vi "SP_Production_Count_DayWise_1.vi"(8 "error in (no error)":errorcluster) -> (0 "error out":errorcluster)   [LabVIEW 2017]
uses:
  <vilib>/Math Plots/3D Math Plots/3D Pie/3D Pie XCtrl/3D Pie.xctl
  <vilib>/addons/database/Connection.llb/DB Tools Open Connec (Path).vi
  <vilib>/addons/database/Connection.llb/Conn Execute.vi
  <vilib>/addons/database/Recordset.llb/Rec Fetch Recordset Data (R).vi
  <vilib>/addons/database/Recordset.llb/Rec Destroy - Connection.vi
  <vilib>/Math Plots/3D Math Plots/3D Pie/3D Pie Datatype/Public/Plot Helper (Vector).vi
  <vilib>/addons/database/NI_Database_API.lvlib
  <vilib>/Math Plots/3D Math Plots/3D Pie/3D Pie Datatype/3D Pie Datatype.lvclass
panel:
  out "Station size":i32
  in  "Tab Control":enum32{"Data", "Graph"}(tab)
  out "Table":string[][](table)
  out "3D Pie":refnum<class "3D Plot Datatype.lvclass">[](xcontrol)
  in  "To Date":timestamp format="%<%Y-%m-%d>T"
  out "Station Count":i32
  in  "Cancel Button - Archive":bool
  in  "Download 2":bool
  in  "Get Rport 2":bool
  in  "Shift":string(combo)
  in  "Station":string(combo)
  in  "From Date":timestamp format="%<%Y-%m-%d>T"
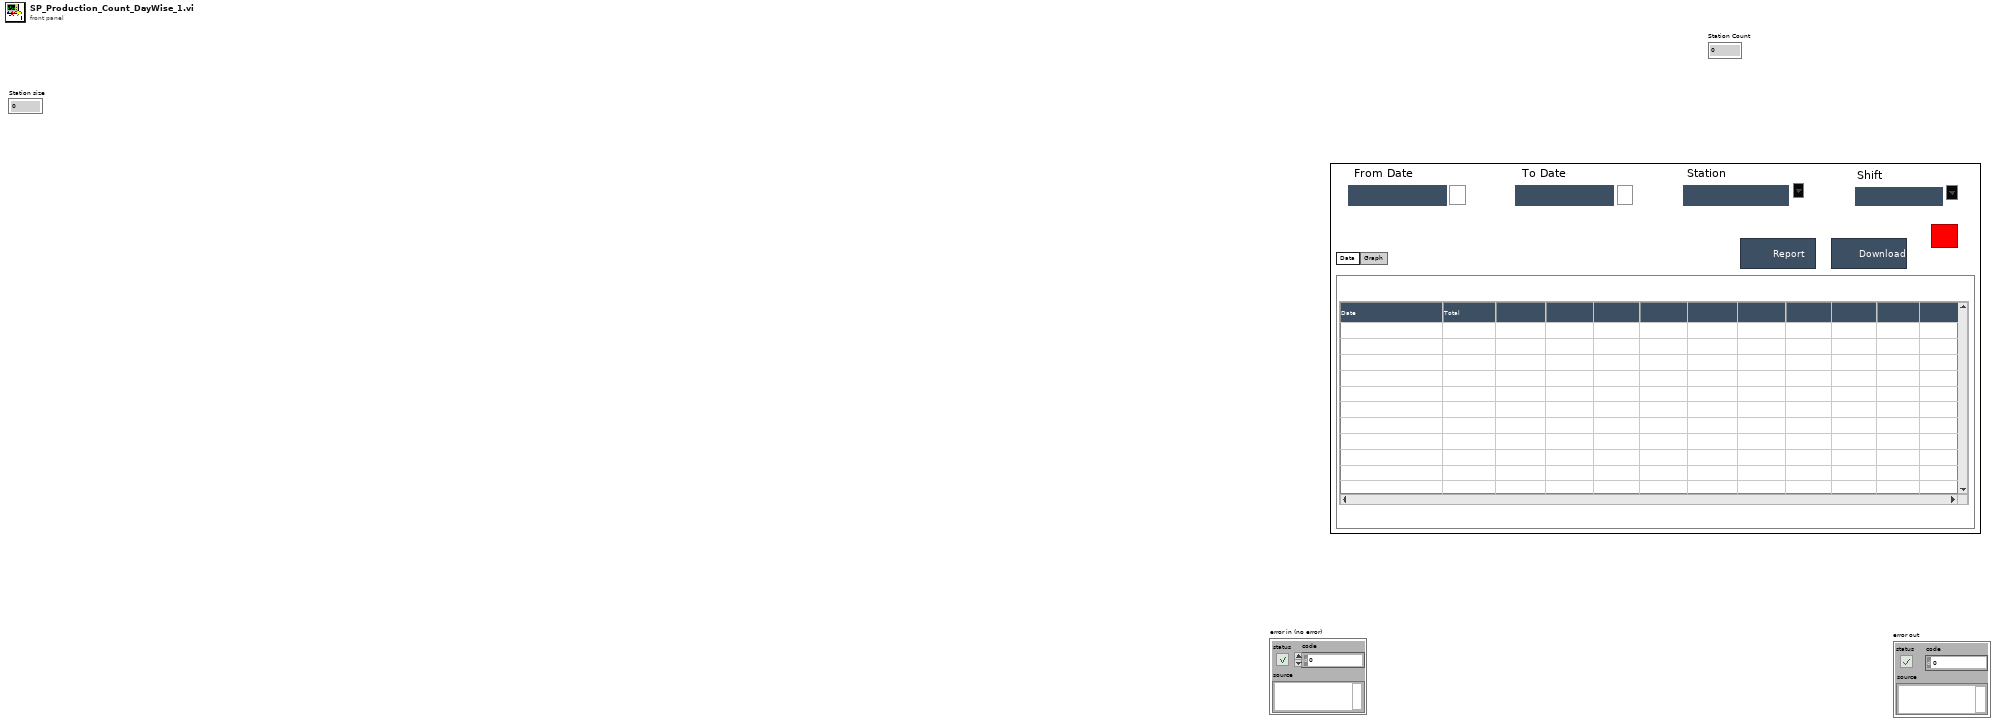
[diagram p1: front panel]
types:
  T1 = typedef "NI_Database_API.lvlib/Conn ObjectReference.ctl" = refnum<k1>
  T2 = typedef "NI_Database_API.lvlib/Rec ObjectReference.ctl" = refnum<k1>
  T3 = enum32{"invalid app kind", "Development System", "Run Time System", "Student Edition", "Embedded LabVIEW", "Evaluation", "Custom"}
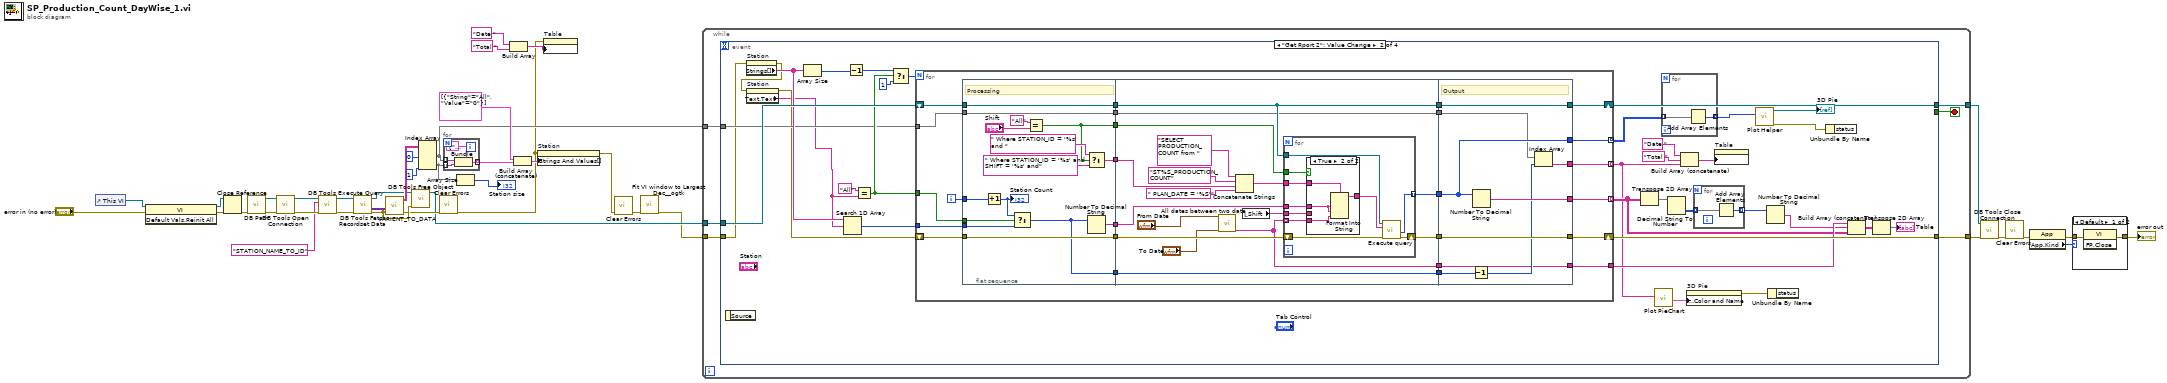
[diagram p0: block diagram]
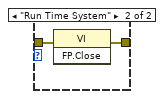
[diagram p2: hidden frame]
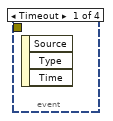
[diagram p3: hidden frame]
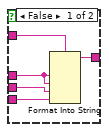
[diagram p4: hidden frame]
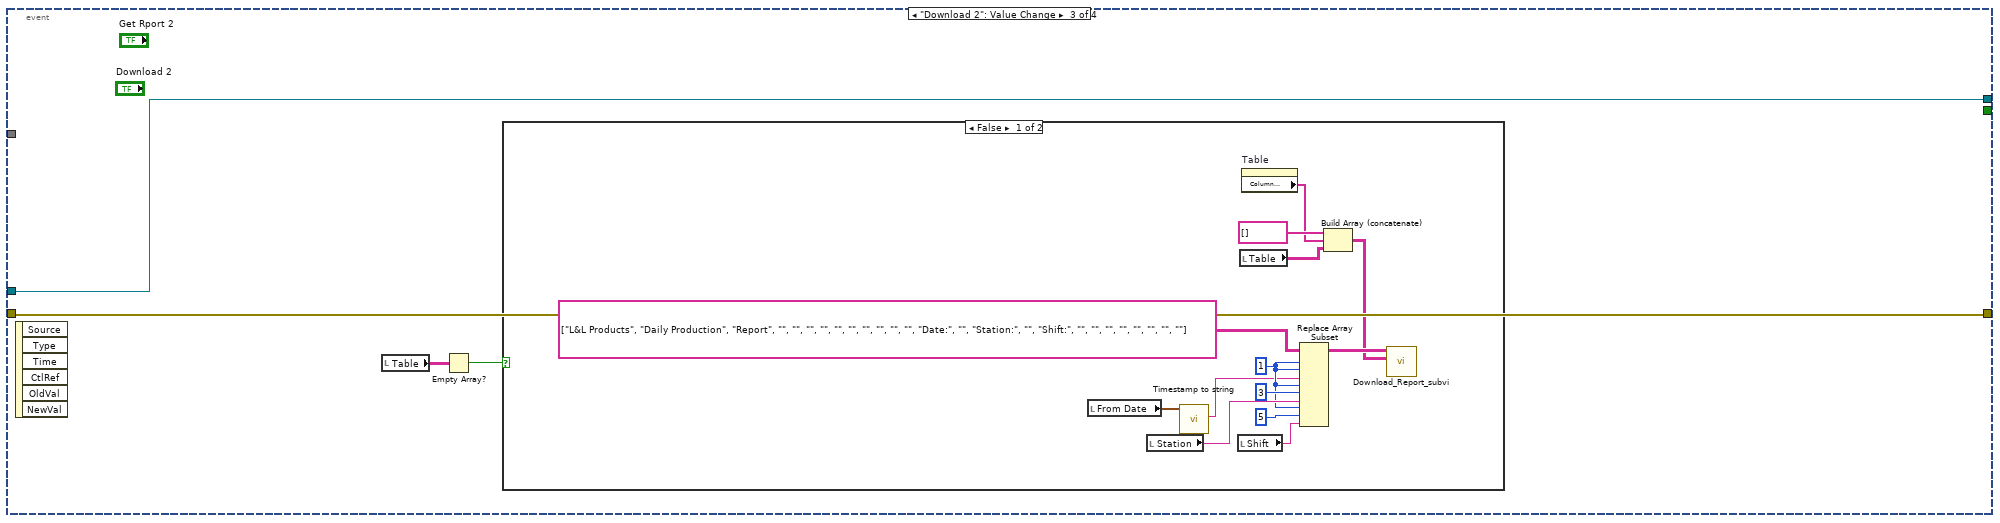
[diagram p5: hidden frame]
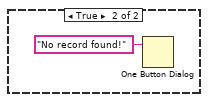
[diagram p6: hidden frame]
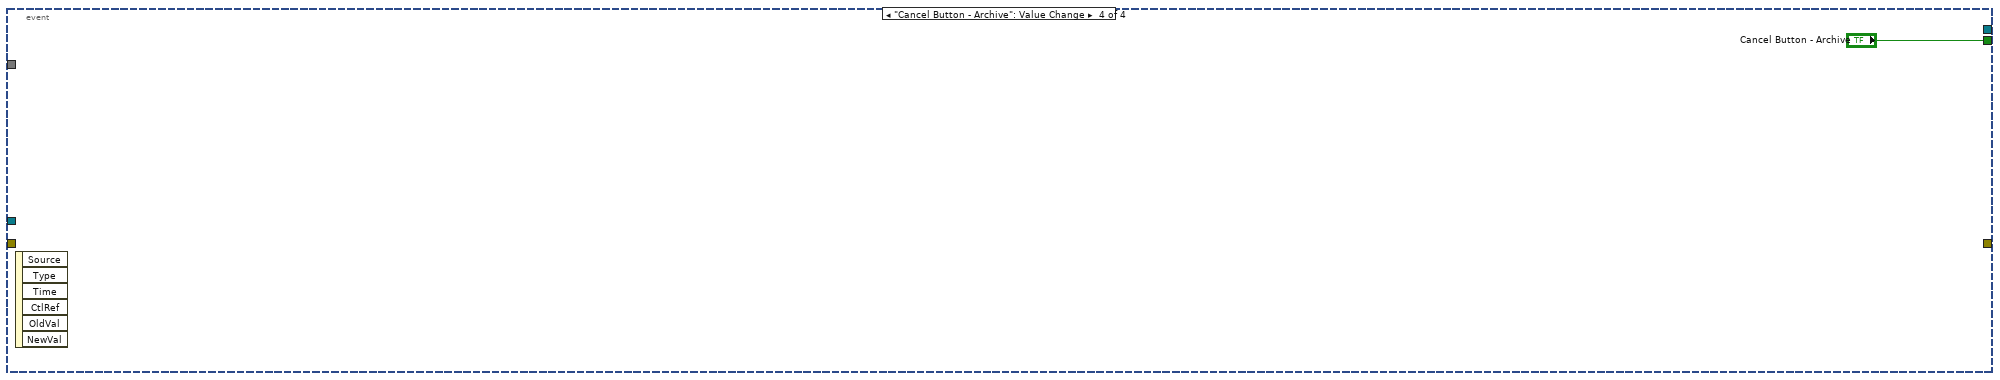
[diagram p7: hidden frame]
diagram:
  n1 = control-ref of="This VI"() -> (w32:refnum<vi>)
  n2 = invoke class="VI" method="Default Vals.Reinit All"(reference=w32, error in="error in (no error)") -> (reference out=w30:refnum<vi>, error out=w31:errorcluster)  [unwired: 1 in, 1 out]
  n3 = Close Reference(reference=w30, error in (no error)=w31) -> (error out=w29:errorcluster)
  n4 = call "DB Path.vi"("error in"=w29) -> ("error out"=w28:errorcluster, "DB Path"=w27:path)  [unwired: 9 in]
  n5 = call-poly <vilib>:"DB Tools Open Connection.vi"("error in (no error)"=w28, "connection information"=w27) -> ("error out"=w16:errorcluster, "connection reference"=w17:T1)  [unwired: 6 in]
  n6 = call-poly <vilib>:"DB Tools Execute Query.vi"("error in (no error)"=w16, "SQL query"="STATION_NAME_TO_ID", "connection reference"=w17) -> ("error out"=w25:errorcluster, "recordset reference"=w26:T2)  [unwired: 5 in]
  n7 = call-poly <vilib>:"DB Tools Fetch Recordset Data.vi"("error in (no error)"=w25, "recordset reference"=w26) -> ("error out"=w20:errorcluster, "recordset data"=w24:variant[][], "recordset reference out"=w18:T2)  [unwired: 3 in]
  n8 = call "VARIENT_TO_DATA.vi"("data"=w24, "error in (no error)"=w20) -> ("Table"=w21:string[][], "error out"=w19:errorcluster)  [unwired: 7 in]
  n9 = call-poly <vilib>:"DB Tools Free Object.vi"("error in (no error)"=w20, "recordset reference"=w18) -> ("connection reference"=w9:T1)  [unwired: 8 in, 1 out]
  n10 = Index Array(array=w21, index (col) #1=0 ("index (row)"), index (col) #2=1 ("index (col)")) -> (element #1=w5:string[], element #2=w11:string[])  [unwired: 2 in]
  n11 = call <vilib>:"Clear Errors.vi"("error in (no error)"=w19) -> ("error out"=w1:errorcluster)  [unwired: 5 in, 1 out]
  n12 = for {
    tunnel: w5 -> [w44] mode=indexing
    tunnel: w11 -> [w43] mode=indexing
    tunnel: [w41] -> w12 mode=indexing
    n13 = Bundle(cluster=cluster{"String":string, "Value":string} {"String"="", "Value"=""}, "String"=w44, "Value"=w43) -> (w41:cluster{"String":string, "Value":string})
  }
  n14 = Array Size(array=w11) -> (size(s)=→"Station size":i32)
  n15 = Build Array("Date ", "Total ") -> (w2:string[])
  n16 = Build Array (concatenate)(cluster{"String":string, "Value":string}[] [{"String"="All", "Value"="0"}] ("array"), w12) -> (w14:cluster{"String":string, "Value":string}[])
  n17 = property on="Station" class="CmbBox"(error in=w1, "Strings And Values[]"=w14) -> (error out=w7:errorcluster)  [unwired: 1 in, 1 out]
  n18 = property on="Table" class="Tbl (strict)"(error in=w1, "Column Headers[]"=w2) -> ()  [unwired: 1 in, 2 out]
  n19 = call <vilib>:"Clear Errors.vi"("error in (no error)"=w7) -> ("error out"=w8:errorcluster)  [unwired: 5 in, 1 out]
  n20 = call <userlib>:"Fit VI window to Largest Dec__ogtk.vi"("error in (no error)"=w8) -> ("error out"=w6:errorcluster)  [unwired: 5 in, 1 out]
  n21 = while {
    tunnel: w6 -> [w47]
    tunnel: w9 -> [w46]
    tunnel: [w49] -> w35
    tunnel: [w48] -> w34
    tunnel: w5 -> [w45]
    stop <- w50 stop-if-true
    n22 = event shown="[1] \"Get Rport 2\": Value Change" {
      selector: _ -> [_ _ _ _]
      dyn-events: _ -> [_ _ _ _]
      timeout: _ -> [_ _ _ _]
      tunnel: w46 -> [_ w84 w177 _]
      tunnel: [_ _ _ "Cancel Button - Archive"] -> w50
      tunnel: [_ w82 w176 _] -> w49
      tunnel: [_ w83 w177 _] -> w48
      tunnel: w47 -> [_ w53 w176 _]
      tunnel: w45 -> [_ w55 _ _]
      event Timeout {
        n23 = event-data() -> ()  [unwired: 1 in, 3 out]
      }
      event "Get Rport 2": Value Change {
        n24 = event-data() -> ()  [unwired: 1 in, 1 out]
        n25 = property on="Station" class="CmbBox"(error in=w53) -> (error out=w54:errorcluster, "Strings[]"=w63:string[])  [unwired: 1 in, 1 out]
        n26 = property on="Station" class="CmbBox"(error in=w54) -> (error out=w52:errorcluster, "Text.Text"=w51:string)  [unwired: 1 in, 1 out]
        n27 = Array Size(array=w63) -> (size(s)=w78:i32)
        n28 = Search 1D Array(1D array=w63, element=w51) -> (index of element=w75:i32)  [unwired: 1 in]
        n29 = Decrement(x=w78) -> (x-1=w77:i32)
        n30 = Equal?(x="All", y=w51) -> (x = y?=w76:bool)
        n31 = Select(t=w77, s=w76, f=1) -> (s? t:f=w80:i32)
        n32 = for {
          N: w80 -> [_]
          shift-right: [w106] -> w83
          shift-left: w84 -> [w113]
          shift-right: [w107] -> w82
          shift-left: w52 -> [w112]
          tunnel: w76 -> [w111]
          tunnel: w75 -> [w110]
          tunnel: [w108] -> w57 mode=indexing
          tunnel: [w98] -> w68 mode=indexing
          tunnel: [w97] -> w71
          tunnel: [w92] -> w59 mode=indexing
          tunnel: w55 -> [w89]
          i -> [w109]
          n33 = flat-sequence {
            tunnel: [w125] -> w105
            tunnel: [w126] -> w103
            tunnel: [w128] -> w101
            tunnel: [w127] -> w100
            tunnel: w109 -> [w120]
            tunnel: w110 -> [w121]
            tunnel: w111 -> [w122]
            tunnel: w112 -> [w125]
            tunnel: w113 -> [w126]
            tunnel: [w116] -> w95
            tunnel: [w115] -> w93
            tunnel: [w114] -> w90
            tunnel: w89 -> [w114]
            tunnel: w105 -> [w138]
            tunnel: [w137] -> w104
            tunnel: w103 -> [w139]
            tunnel: [w139] -> w102
            tunnel: w101 -> [w143]
            tunnel: w100 -> [w135]
            tunnel: [w136] -> w99
            tunnel: [w134] -> w96
            tunnel: w95 -> [w131]
            tunnel: [w130] -> w94
            tunnel: w93 -> [w130]
            tunnel: [w129] -> w91
            tunnel: w90 -> [w129]
            tunnel: [w169] -> w108
            tunnel: w104 -> [w171]
            tunnel: [w171] -> w107
            tunnel: [w173] -> w106
            tunnel: w102 -> [w173]
            tunnel: w99 -> [w167]
            tunnel: [w172] -> w98
            tunnel: [w166] -> w97
            tunnel: w96 -> [w166]
            tunnel: w94 -> [w170]
            tunnel: [w167] -> w92
            tunnel: w91 -> [w165]
            frame #0 {
              # "Processing"
              n34 = Increment(x=w120) -> (x+1=w119:i32)
              "Station Count" <- w119
              n35 = Select(t=w119, s=w122, f=w121) -> (s? t:f=w115:i32)
              n36 = Equal?(x="All", y="Shift") -> (x = y?=w116:bool)
              n37 = Select(t=" Where STATION_ID = '%s' and " ("format string"), s=w116, f=" Where STATION_ID = '%s' and SHIFT = '%s' and" ("format string")) -> (s? t:f=w128:string)
              n38 = Number To Decimal String(number=w115) -> (decimal integer string=w127:string)  [unwired: 1 in]
            }
            frame #1 {
              n39 = call "All dates between two date.vi"("To Date"="To Date", "From Date"="From Date") -> ("All Days (String)"=w134:string[])  [unwired: 8 in, 1 out]
              n40 = Concatenate Strings("SELECT  PRODUCTION_COUNT from " ("format string"), "ST%S_PRODUCTION_COUNT", w143, " PLAN_DATE = '%S'" ("string")) -> (w141:string)
              n41 = local read "Shift"() -> (w140:string)
              n42 = for {
                tunnel: w131 -> [w155]
                tunnel: w141 -> [w154]
                tunnel: w135 -> [w153]
                tunnel: w140 -> [w152]
                tunnel: w134 -> [w151] mode=indexing
                tunnel: w139 -> [w149]
                shift-right: [w147] -> w137
                shift-left: w138 -> [w148]
                tunnel: [w146] -> w136 mode=indexing
                n43 = case shown="True" w155 {
                  tunnel: w154 -> [w160 w164]
                  tunnel: w153 -> [w159 w163]
                  tunnel: w152 -> [w158 _]
                  tunnel: w151 -> [w157 w162]
                  tunnel: [w156 w161] -> w150
                  frame False {
                    n44 = Format Into String(format string=w160, w159, w159, w158, w157) -> (resulting string=w156:string)  [unwired: 2 in, 1 out]
                  }
                  frame True {
                    n45 = Format Into String(format string=w164, w163, w163, w162) -> (resulting string=w161:string)  [unwired: 2 in, 1 out]
                  }
                }
                n46 = call "Execute query.vi"("error in (no error)"=w148, "String"=w150, "connection reference"=w149) -> ("error out"=w147:errorcluster, "Production Count"=w146:i32)  [unwired: 3 in, 4 out]
              }
            }
            frame #2 {
              # "Output"
              n47 = Decrement(x=w170) -> (x-1=w168:i32)
              n48 = Number To Decimal String(number=w167) -> (decimal integer string=w172:string[])  [unwired: 1 in]
              n49 = Index Array(array=w165, index=w168) -> (element=w169:string)
            }
          }
        }
        n50 = Transpose 2D Array(2D array=w68) -> (transposed array=w67:string[][])
        n51 = call "Plot PieChart.vi"("Label"=w57) -> ("Labelling"=w58:cluster{dbl, "String":string}[])  [unwired: 10 in]
        n52 = for {
          tunnel: w59 -> [w86] mode=indexing
          tunnel: [w85] -> w60 mode=indexing
          n53 = Add Array Elements(numeric array=w86) -> (sum=w85:i32)
        }
        n54 = Decimal String To Number(string=w67) -> (number=w66:i32[][])  [unwired: 2 in, 1 out]
        n55 = Build Array (concatenate)("Date ", "Total ", w57) -> (w74:string[])
        n56 = property on="3D Pie" class="3D Pie (strict)"("Plot Specific:Color and Name"=w58) -> (error out=w56:errorcluster)  [unwired: 2 in, 1 out]
        n57 = for {
          tunnel: w66 -> [w88] mode=indexing
          tunnel: [w87] -> w65 mode=indexing
          n58 = Add Array Elements(numeric array=w88) -> (sum=w87:i32)
        }
        n59 = property on="Table" class="Tbl (strict)"("Column Headers[]"=w74) -> ()  [unwired: 2 in, 2 out]
        n60 = call-poly <vilib>:"Plot Helper.vi"("x vector"=w60) -> ("error out"=w61:errorcluster, "3D Plot lvclass Array out"=→"3D Pie":refnum<class "3D Plot Datatype.lvclass">[])  [unwired: 2 in, 7 out]
        n61 = Number To Decimal String(number=w65) -> (decimal integer string=w64:string[])  [unwired: 1 in]
        n62 = Unbundle By Name(w56) -> ()  [unwired: 1 out]
        n63 = Unbundle By Name(w61) -> ()  [unwired: 1 out]
        n64 = Build Array (concatenate)(w71, w64, w68) -> (w73:string[][])
        n65 = Transpose 2D Array(2D array=w73) -> (transposed array=→"Table":string[][])
      }
      event "Download 2": Value Change {
        n66 = event-data() -> ()  [unwired: 1 in, 6 out]
        n67 = local read "Table"() -> (w175:string[][])
        n68 = Empty Array?(array=w175) -> (empty?=w174:bool)
        n69 = case shown="False" w174 {
          frame False {
            w186 = 1 ("index (row)")
            n70 = local read "From Date"() -> (w183:timestamp)
            n71 = local read "Station"() -> (w187:string)
            n72 = call "Timestamp to string.vi"("time stamp"=w183) -> ("Date"=w182:string)  [unwired: 8 in, 2 out]
            n73 = local read "Shift"() -> (w184:string)
            n74 = local read "Table"() -> (w181:string[][])
            n75 = property on="Table" class="Tbl (strict)"() -> ("Column Headers[]"=w178:string[])  [unwired: 2 in, 2 out]
            n76 = Replace Array Subset(array=string[][] [["L&L Products", "Daily Production", "Report", "", "", "", "", "", "", "", "", "", ""], ["Date:", "", "Station:", "", "Shift:", "", "", "", "", "", "", "", ""]] ("Column Header Strings[]"), new element #1=w182, index (row) #1=w186, index (col) #1=w186, new element #2=w187, index (row) #2=w186, index (col) #2=3 ("disabled index (col)"), new element #3=w184, index (row) #3=w186, index (col) #3=5 ("disabled index (col)")) -> (w189:string[][])
            n77 = Build Array (concatenate)(string[] [] ("element"), w178, w181) -> (w180:string[][])
            n78 = call "Download_Report_subvi.vi"("Value"=w180, "Column Header Strings[]"=w189) -> ()  [unwired: 9 in, 1 out]
          }
          frame True {
            n79 = One Button Dialog(message="No record found!") -> ()  [unwired: 1 in, 1 out]
          }
        }
      }
      event "Cancel Button - Archive": Value Change {
        n80 = event-data() -> ()  [unwired: 1 in, 6 out]
      }
    }
  }
  n81 = call <vilib>:"DB Tools Close Connection.vi"("error in (no error)"=w35, "connection reference"=w34) -> ("error out"=w37:errorcluster)  [unwired: 5 in]
  n82 = call <vilib>:"Clear Errors.vi"("error in (no error)"=w37) -> ("error out"=w36:errorcluster)  [unwired: 5 in, 1 out]
  n83 = property class="App"(error in=w36) -> (error out=w38:errorcluster, "App.Kind"=w39:T3)  [unwired: 1 in, 1 out]
  n84 = case shown="Default" w39 {
    tunnel: w38 -> [w194 w196]
    tunnel: [w193 w195] -> w33
    frame Default {
      n85 = invoke class="VI" method="FP.Close"(error in=w194) -> (error out=w193:errorcluster)  [unwired: 2 in, 2 out]
    }
    frame "Run Time System" {
      n86 = invoke class="VI" method="FP.Close"(error in=w196) -> (error out=w195:errorcluster)  [unwired: 2 in, 2 out]
    }
  }
  "error out" <- w33
